vi "Pigeon_IMU.vi"(10 "T/F":bool) -> (2 "Yaw":dbl)   [LabVIEW 2020]
uses:
  <vilib>/Rock Robotics/WPI/ThirdParty/Phoenix-LabVIEW/Pigeon IMU/CTRE_PigeonIMU_GetYPR.vi
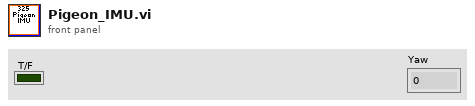
[diagram p1: front panel]
types:
  T1 = typedef "CTRE_PigeonIMU_DeviceRef.ctl" = cluster{"DeviceStatus":errorcluster, "Device Number":u8, "Type":T2, "Device ID":u32, "Handle":u64, "UsageFrame":u32, "Library Path":path}
  T2 = typedef "CTRE_PigeonIMU_ConnectionType.ctl" = u32
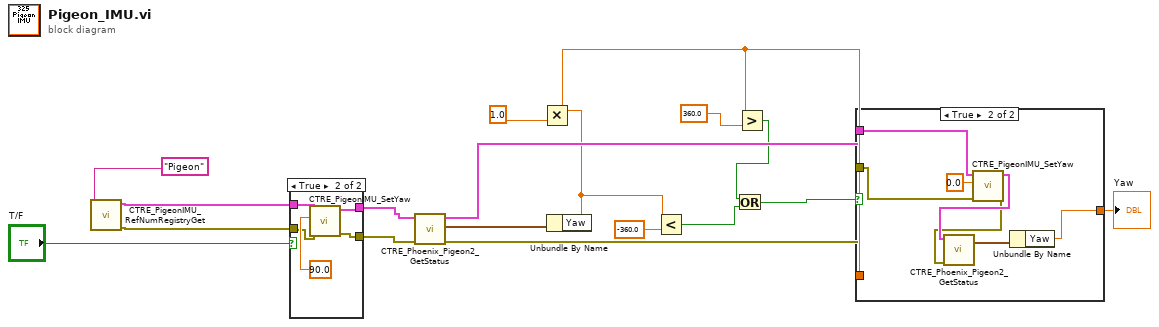
[diagram p0: block diagram]
diagram:
  n1 = call <vilib>:"CTRE_PigeonIMU_RefNumRegistryGet.vi"("refnum name"="Pigeon") -> ("error out"=w17:errorcluster, "PigeonIMUDevRef"=w18:T1)  [unwired: 9 in]
  n2 = case shown="True" "T/F" {
    tunnel: w18 -> [w20 w24]
    tunnel: [w20 w23] -> w13
    tunnel: w17 -> [w19 w21]
    tunnel: [w19 w22] -> w12
    frame False {
    }
    frame True {
      n3 = call <vilib>:"CTRE_PigeonIMU_SetYaw.vi"("error in (no error)"=w21, "Value"=90.0, "PigeonIMUDevRef"=w24) -> ("error out"=w22:errorcluster, "PigeonIMUDevRef"=w23:T1)  [unwired: 7 in]
    }
  }
  n4 = call-poly <vilib>:"CTRE_Phoenix_Pigeon2_GetStatus.vi"("error in (no error)"=w12, "PigeonIMUDevRef"=w13) -> ("error out"=w8:errorcluster, "Yaw Pitch Roll"=w14:cluster{"Yaw":dbl, "Pitch":dbl, "Roll":dbl}, "PigeonIMUDevRef"=w9:T1)  [unwired: 7 in]
  n5 = Unbundle By Name(w14) -> ("Yaw"=w5:dbl)
  n6 = Multiply(x=w5, y=1.0) -> (x*y=w10:dbl)
  n7 = Less?(x=w5, y=-360.0) -> (x < y?=w6:bool)
  n8 = Greater?(x=w10, y=360.0) -> (0:w7:bool)
  n9 = Or(x=w7, y=w6) -> (x .or. y?=w3:bool)
  n10 = case shown="True" w3 {
    tunnel: [w26 w27] -> w1
    tunnel: w10 -> [w26 _]
    tunnel: w9 -> [_ w33]
    tunnel: w8 -> [_ w32]
    frame False {
    }
    frame True {
      n11 = call <vilib>:"CTRE_PigeonIMU_SetYaw.vi"("error in (no error)"=w32, "Value"=0.0, "PigeonIMUDevRef"=w33) -> ("error out"=w28:errorcluster, "PigeonIMUDevRef"=w29:T1)  [unwired: 7 in]
      n12 = call-poly <vilib>:"CTRE_Phoenix_Pigeon2_GetStatus.vi"("error in (no error)"=w28, "PigeonIMUDevRef"=w29) -> ("Yaw Pitch Roll"=w30:cluster{"Yaw":dbl, "Pitch":dbl, "Roll":dbl})  [unwired: 7 in, 2 out]
      n13 = Unbundle By Name(w30) -> ("Yaw"=w27:dbl)
    }
  }
  "Yaw" <- w1
